vi "create.vi"(8 "error in (no error)":errorcluster, 11 "Type":T1=enum."DMM_NI") -> (0 "error out":errorcluster, 3 "Multimeter.lvclass":refnum<class "Multimeter.lvclass">)   [LabVIEW 2023, in "sweDmm.lvlib"]
doc: "Create New DMM Object."
uses:
  sweDmm.lvlib
  Data/DmmTypes.ctl
  Multimeter.lvclass
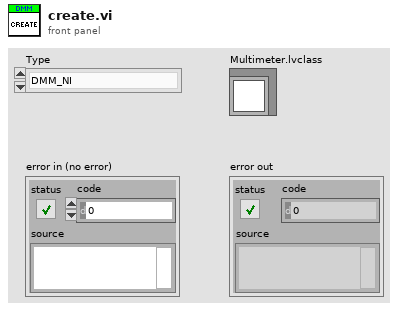
[diagram p1: front panel]
types:
  T1 = typedef "sweDmm.lvlib/DmmTypes.ctl" = enum16{"Simulated", "DMM_NI", "DMM_Keysight"}
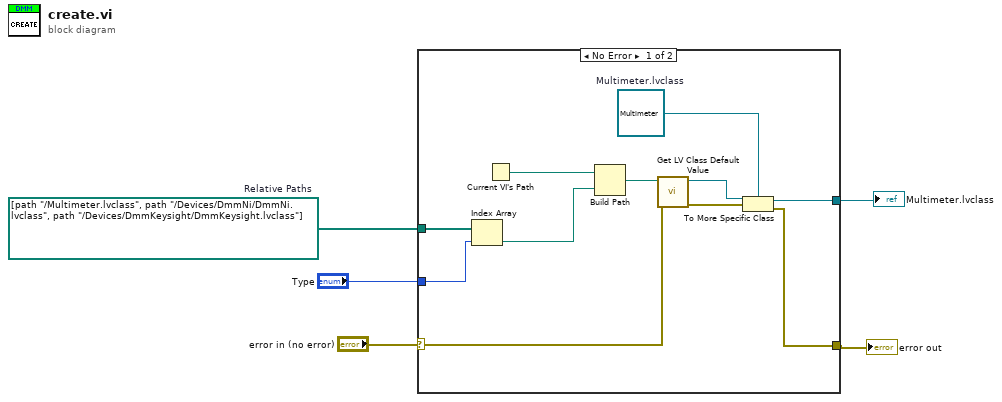
[diagram p0: block diagram]
diagram:
  w1 = path[] [path "../Multimeter.lvclass", path "../Devices/DmmNi/DmmNi.lvclass", path "../Devices/DmmKeysight/DmmKeysight.lvclass"]  # Relative Paths
  n1 = case shown="No Error" "error in (no error)" {
    selector: "error in (no error)" -> [w15 w17]
    tunnel: [w13 _] -> w5
    tunnel: w1 -> [w12 _]
    tunnel: "Type" -> [w10 _]
    tunnel: [w7 w17] -> w4
    frame No Error {
      w6 = refnum<class "Multimeter.lvclass"> refnum  # Multimeter.lvclass
      n2 = Index Array "Index Array"(array=w12, index=w10) -> (element=w11:path)
      n3 = Current VI's Path() -> (path=w16:path)
      n4 = Build Path(base path=w16, name or relative path=w11) -> (appended path=w14:path)
      n5 = call <vilib>:"Get LV Class Default Value.vi"("error in (no error)"=w15, "class path"=w14) -> ("error out"=w9:errorcluster, "object"=w8:refnum<class>)  [unwired: 8 in]
      n6 = To More Specific Class(target class=w6, reference=w8, error in=w9) -> (specific class reference=w13:refnum<class "Multimeter.lvclass">, error out=w7:errorcluster)
    }
    frame Error {
    }
  }
  "error out" <- w4
  "Multimeter.lvclass" <- w5
